vi "_db(lvlibp).vi"(7 "command":T1(ring), 8 "error in (no error)":errorcluster, 10 "db in":refnum<k1>, 11 "name":string) -> (0 "error out":errorcluster, 1 "created new?":bool, 3 "db out":refnum<k1>, 4 "info":cluster{"db":refnum<k1>, "Count":i32}, 6 "db list":string[](array[string]))   [LabVIEW 2017, in "TagDB.lvlib"]
doc: "[Covers: REQ_TAGDB_NAMEDDB]"
uses:
  TagDB.lvlib
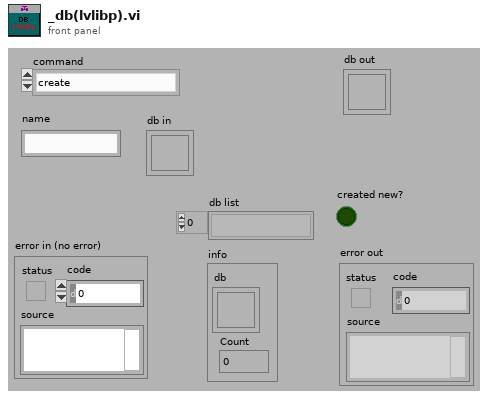
[diagram p1: front panel]
types:
  T1 = enum16{"create", "destroy", "cleanUp", "list", "get info", "force destroy"}
  T2 = cluster{"inputs":cluster{"command":enum16{"create", "destroy", "cleanUp", "list", "get info", "force destroy"}, "name":string, "db in":refnum<k1>}, "ReturnQ":refnum<queue>, "WatchdogQueue":refnum<queue>}
  T3 = cluster{"db out":refnum<k1>, "db list":string[], "info":cluster{"db":refnum<k1>, "Count":i32}, "created new?":bool, "error out":errorcluster}
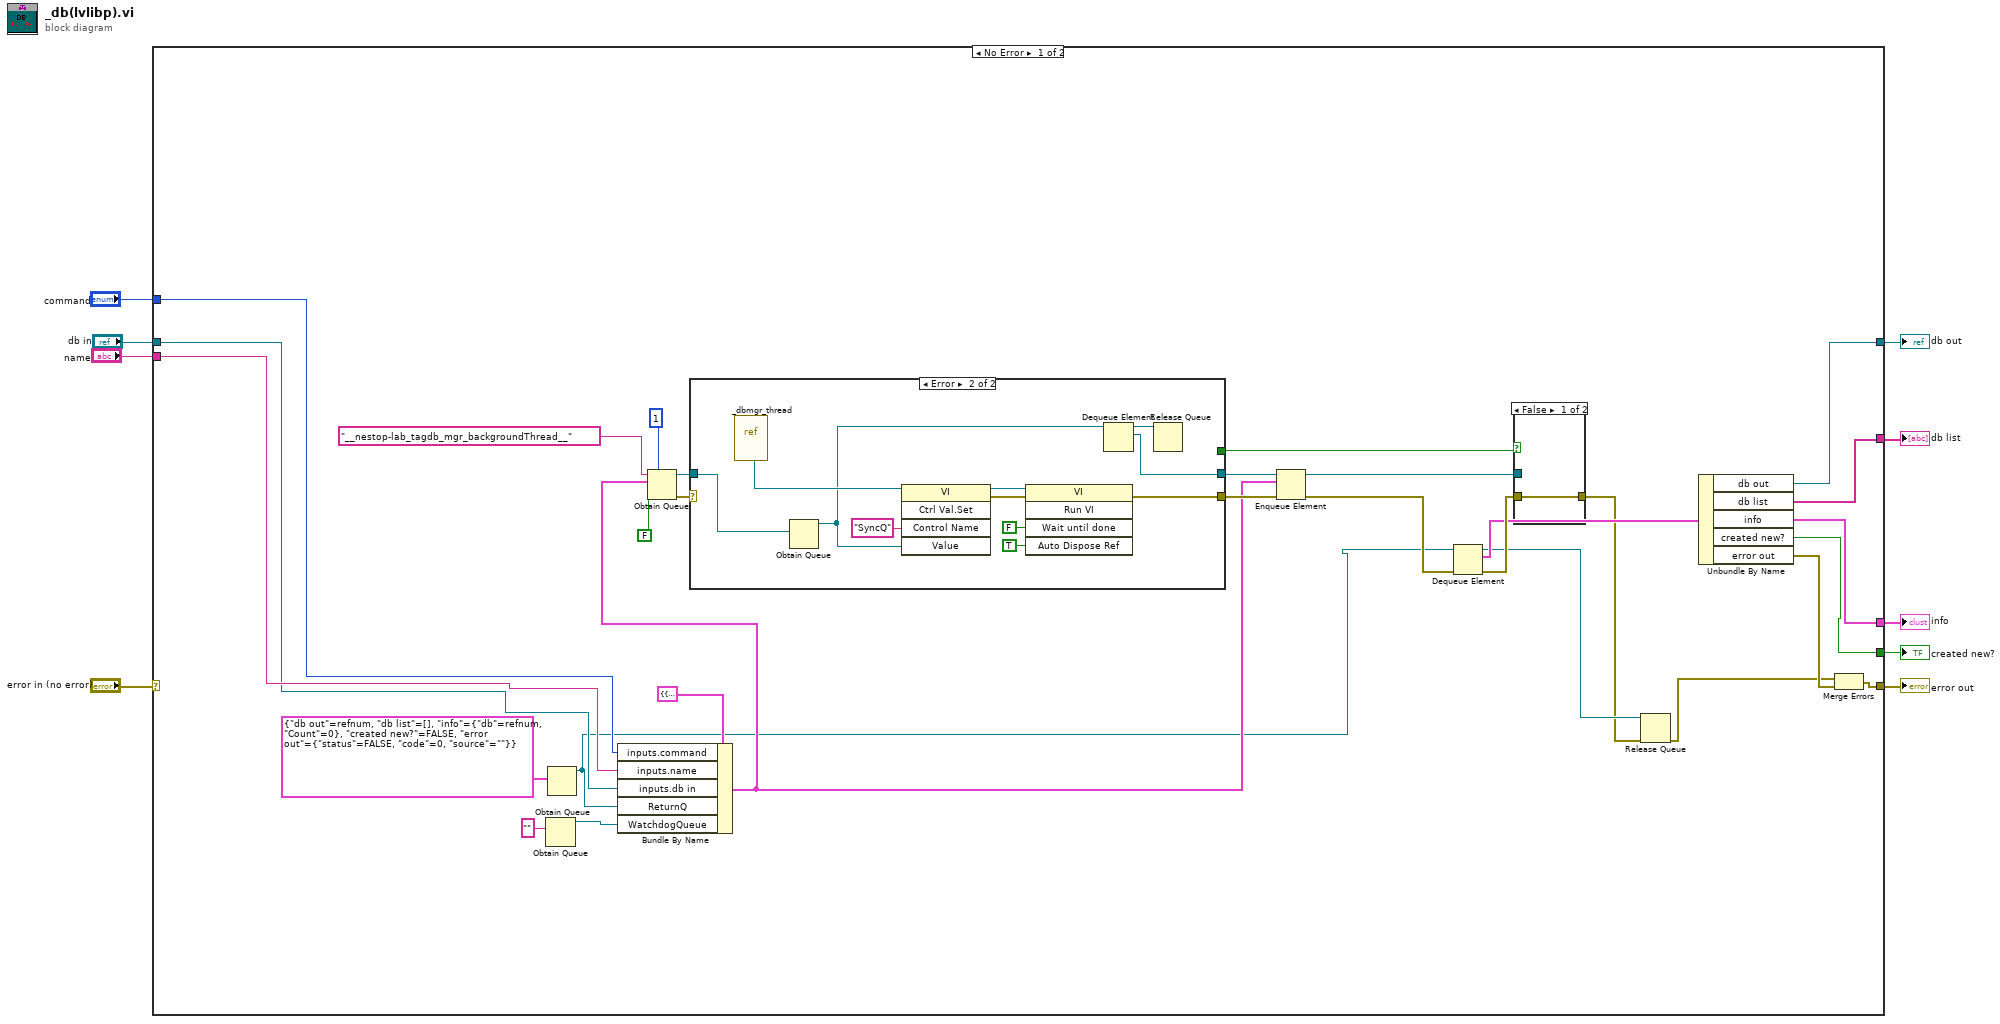
[diagram p0: block diagram]
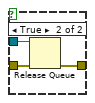
[diagram p2: hidden frame]
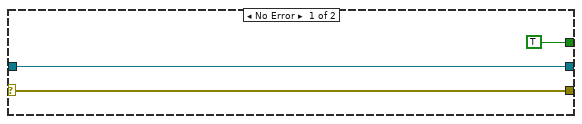
[diagram p3: hidden frame]
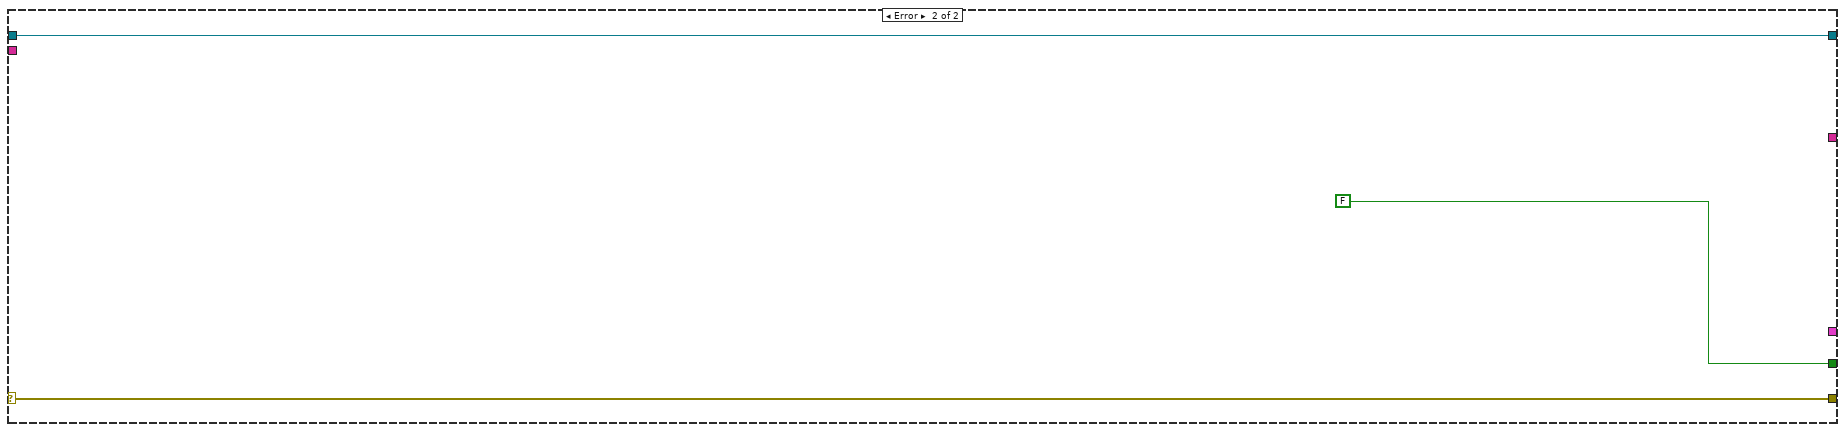
[diagram p4: hidden frame]
diagram:
  n1 = case shown="No Error" "error in (no error)" {
    selector: "error in (no error)" -> [_ w60]
    tunnel: [w19 w60] -> w6
    tunnel: [w21 FALSE ("created new?")] -> w5
    tunnel: "name" -> [w13 _]
    tunnel: "command" -> [w14 _]
    tunnel: "db in" -> [w12 w58]
    tunnel: [w24 w58] -> w3
    tunnel: [w23 _] -> w2
    tunnel: [w22 _] -> w1
    frame No Error {
      n2 = Obtain Queue(element data type="" ("name (unnamed)")) -> (queue out=w37:refnum<queue>)  [unwired: 4 in, 2 out]
      n3 = Obtain Queue(element data type=T3 {"db out"=refnum, "db list"=[], "info"={"db"=refnum, "Count"=0}, "created new?"=FALSE, "error out"={"status"=FALSE, "code"=0, "source"=""}}) -> (queue out=w10:refnum<queue>)  [unwired: 4 in, 2 out]
      n4 = Bundle By Name(cluster=T2 {"inputs"={"command"=enum."create", "name"="", "db in"=refnum}, "ReturnQ"=refnum, "WatchdogQueue"=refnum}, "inputs.command"=w14, "inputs.name"=w13, "inputs.db in"=w12, "ReturnQ"=w10, "WatchdogQueue"=w37) -> (w11:T2)
      n5 = Obtain Queue(max queue size (-1, unlimited)=1, name (unnamed)="__nestop-lab_tagdb_mgr_backgroundThread__", element data type=w11, create if not found? (T)=FALSE) -> (queue out=w29:refnum<queue>, error out=w36:errorcluster)  [unwired: 1 in, 1 out]
      n6 = case shown="Error" w36 {
        selector: w36 -> [w46 _]
        tunnel: [w46 w54] -> w38
        tunnel: w29 -> [w45 w49]
        tunnel: [w45 w48] -> w28
        tunnel: [TRUE _] -> w27
        frame No Error {
        }
        frame Error {
          n7 = vi-ref "_dbmgr_thread.vi"() -> (w57:refnum<vi>)
          n8 = Obtain Queue(element data type=w49) -> (queue out=w51:refnum<queue>)  [unwired: 4 in, 2 out]
          n9 = invoke class="VI" method="Ctrl Val.Set"(reference=w57, "Control Name"="SyncQ", "Value"=w51) -> (reference out=w53:refnum<vi>, error out=w47:errorcluster)  [unwired: 2 in, 3 out]
          n10 = invoke class="VI" method="Run VI"(reference=w53, error in=w47, "Wait until done"=FALSE ("Wait Until Done"), "Auto Dispose Ref"=TRUE ("Auto Dispose Reference")) -> (error out=w54:errorcluster)  [unwired: 1 in, 4 out]
          n11 = Dequeue Element(queue=w51) -> (queue out=w50:refnum<queue>, element=w48:refnum<queue>)  [unwired: 2 in, 2 out]
          n12 = Release Queue(queue=w50) -> ()  [unwired: 2 in, 3 out]
        }
      }
      n13 = Enqueue Element(queue=w28, element=w11, error in (no error)=w38) -> (queue out=w32:refnum<queue>, error out=w39:errorcluster)  [unwired: 1 in, 1 out]
      n14 = Dequeue Element(queue=w10, error in (no error)=w39) -> (queue out=w18:refnum<queue>, element=w25:T3, error out=w31:errorcluster)  [unwired: 1 in, 1 out]
      n15 = case shown="False" w27 {
        tunnel: w32 -> [_ w43]
        tunnel: w31 -> [w40 w42]
        tunnel: [w40 w41] -> w17
        frame False {
        }
        frame True {
          n16 = Release Queue(queue=w43, error in (no error)=w42) -> (error out=w41:errorcluster)  [unwired: 1 in, 2 out]
        }
      }
      n17 = Release Queue(queue=w18, error in (no error)=w17) -> (error out=w16:errorcluster)  [unwired: 1 in, 2 out]
      n18 = Unbundle By Name(w25) -> ("db out"=w24:refnum<k1>, "db list"=w23:string[], "info"=w22:cluster{"db":refnum<k1>, "Count":i32}, "created new?"=w21:bool, "error out"=w20:errorcluster)
      n19 = Merge Errors(w16, w20) -> (w19:errorcluster)
    }
    frame Error {
    }
  }
  "created new?" <- w5
  "error out" <- w6
  "db out" <- w3
  "db list" <- w2
  "info" <- w1
